vi "onListenForNewConnection.vi"(8 "error in (no error)":errorcluster, 9 "timeout (ms)":i32=2000, 11 "Listener":refnum<class "Connection.Collection.lvclass">) -> (0 "error out":errorcluster, 1 "New connection":bool, 2 "timed out":bool, 3 "New Connection":refnum<class "Connection.lvclass">)   [LabVIEW 2013, in "Connection_GOSPL.lvlib" / "Connection.Collection.lvclass"]
uses:
  Connection.Collection.lvclass
  Connection/Connection.lvclass
  Connection.Collection.lvclass/Connection.Collection.ctl
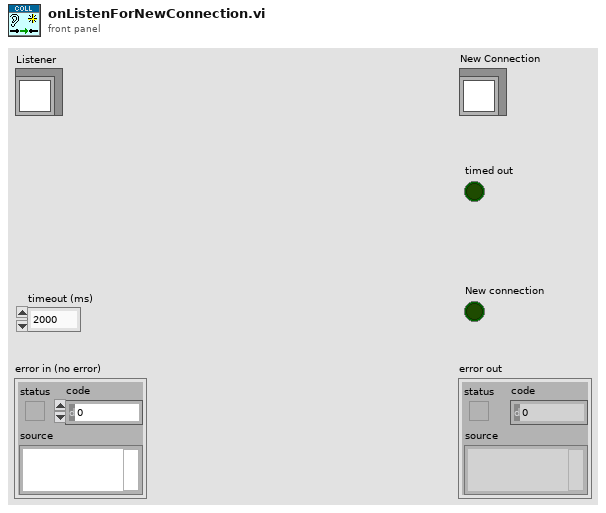
[diagram p1: front panel]
types:
  T1 = typedef "Connection_GOSPL.lvlib/Connection.Collection.lvclass/incoming connection.ctl" = cluster{"Connection":refnum<class "Connection.lvclass">, "error":errorcluster}
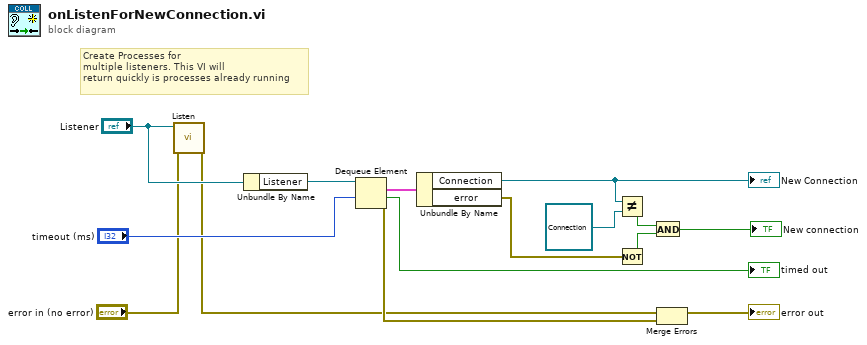
[diagram p0: block diagram]
diagram:
  # "Create Processes for\nmultiple listeners. This VI will\nreturn quickly is processes already running"
  n1 = call "Listen.vi"("error in (no error)"="error in (no error)", "Connection.Collection"="Listener") -> ("error out"=w2:errorcluster)  [unwired: 8 in, 1 out]
  n2 = Unbundle By Name("Listener") -> ("Listener"=w14:refnum<queue>)
  n3 = Dequeue Element(queue=w14, timeout in ms (-1)="timeout (ms)") -> (element=w12:T1, timed out?=→"timed out":bool, error out=w13:errorcluster)  [unwired: 1 in, 1 out]
  n4 = Unbundle By Name(w12) -> ("Connection"=w8:refnum<class "Connection.lvclass">, "error"=w10:errorcluster)
  "New Connection" <- w8
  n5 = Not Equal?(x=w8, y=refnum<class "Connection.lvclass"> refnum ("Connection")) -> (x != y?=w7:bool)
  n6 = Not(x=w10) -> (.not. x?=w6:bool)
  n7 = And(x=w7, y=w6) -> (x .and. y?=→"New connection":bool)
  n8 = Merge Errors(w2, w13) -> (→"error out":errorcluster)
